vi "Get Exposure Mode.vi"(8 "error in (no error)":errorcluster) -> (0 "error out":errorcluster, 2 "exposure mode":T1)   [LabVIEW 2017]
doc: "Returns the current exposure mode.\n\n1= automatic\n0= manual"
uses:
  HighFinesse WS5/Variable Typedefs.llb/Exposure Mode.ctl
  HighFinesse WS5/wlmData.dll
  HighFinesse WS5/HighFinesse WS5.lvlib
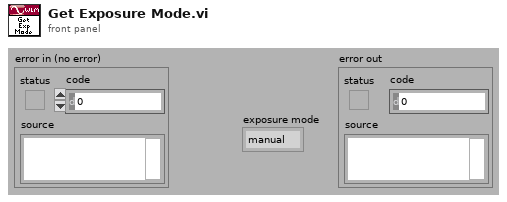
[diagram p1: front panel]
types:
  T1 = typedef "HighFinesse WS5.lvlib/Exposure Mode.ctl" = enum16{"manual", "automatic"}
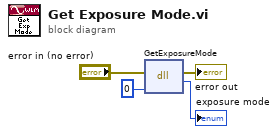
[diagram p0: block diagram]
diagram:
  n1 = dll-call lib="C:/LabVIEW-programs-dev/Instruments/Wavelength meter/HighFinesse WS5/wlmData.dll" fn="GetExposureMode"(error in="error in (no error)", "EM"=u8 0) -> (error out=→"error out":errorcluster, "return type"=→"exposure mode":u8)  [unwired: 3 in, 1 out]
